vi "modeSuperposition_mk.vi"(0 "y_centre (in m; default 0)":dbl step=0.0001 format="%.5f", 1 "modes":T1(array[cluster])=[{"type"=enum."LG mode", "m or L"=-2, "n or p"=0, "weight"=0.7071, "phase"=0.0}, {"type"=enum."LG mode", "m or L"=2, "n or p"=0, "weight"=0.7071, "phase"=0.0}], 2 "beam waist w0 (in m; default 1E-4 = 0.1mm)":dbl=0.0005 format="%.2p", 3 "number of columns in amplitude matrix":i32, 4 "wavelength (in m)":dbl=7.1e-07 format="%#_6p", 5 "number of rows in amplitude matrix":i32, 6 "x_centre (in m; default 0)":dbl step=0.0001 format="%.5f", 8 "represented width & height (in m)":dbl=0.006 format="%#_6p") -> (7 "mode superposition":T2={"amplitude matrix"=array600x600[360000 elements], "number of columns in amplitude matrix"=600, "number of rows in amplitude matrix"=600, "represented width (in m)"=0.006, "represented height (in m)"=0.006, "wavelength (in m)"=7.1e-07})   [LabVIEW 2015]
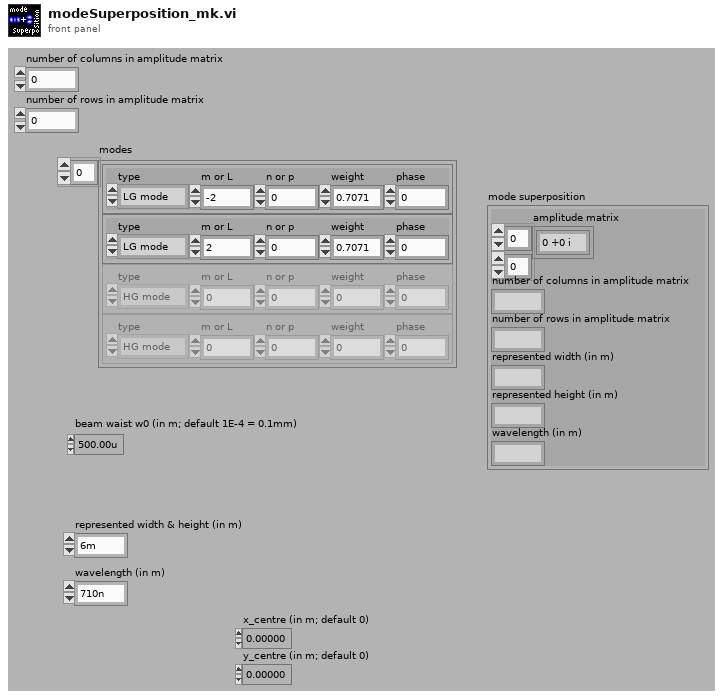
[diagram p1: front panel]
types:
  T1 = cluster{"type":enum16{"HG mode", "LG mode"}, "m or L":i32, "n or p":i32, "weight":dbl, "phase":dbl}[]
  T2 = cluster{"amplitude matrix":cdb[][], "number of columns in amplitude matrix":i32, "number of rows in amplitude matrix":i32, "represented width (in m)":dbl, "represented height (in m)":dbl, "wavelength (in m)":dbl}
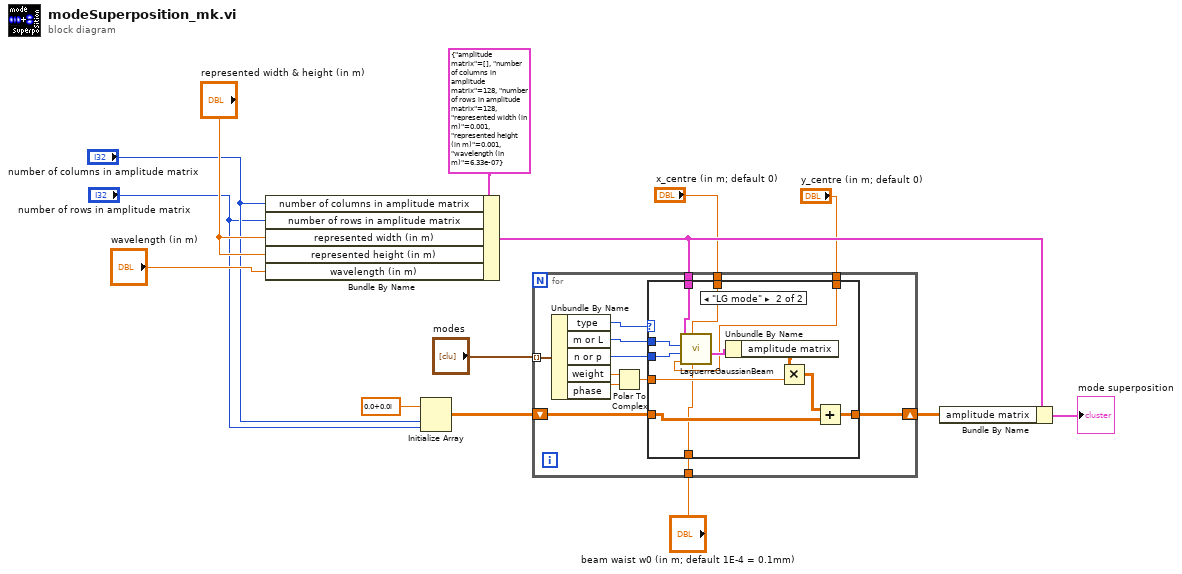
[diagram p0: block diagram]
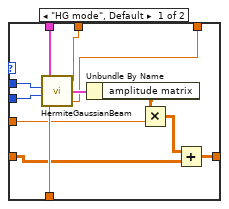
[diagram p2: hidden frame]
diagram:
  n1 = Bundle By Name(cluster=T2 {"amplitude matrix"=[], "number of columns in amplitude matrix"=128, "number of rows in amplitude matrix"=128, "represented width (in m)"=0.001, "represented height (in m)"=0.001, "wavelength (in m)"=6.33e-07} ("beam parameters"), "number of columns in amplitude matrix"="number of columns in amplitude matrix", "number of rows in amplitude matrix"="number of rows in amplitude matrix", "represented width (in m)"="represented width & height (in m)", "represented height (in m)"="represented width & height (in m)", "wavelength (in m)"="wavelength (in m)") -> (w7:T2)
  n2 = Initialize Array(cdb 0.0+0.0i ("element"), "number of columns in amplitude matrix", "number of rows in amplitude matrix") -> (w13:cdb[][])
  n3 = for {
    tunnel: "modes" -> [w27] mode=indexing
    shift-right: [w18] -> w8
    shift-left: w13 -> [w17]
    tunnel: w7 -> [w24]
    tunnel: "beam waist w0 (in m; default 1E-4 = 0.1mm)" -> [w25]
    tunnel: "x_centre (in m; default 0)" -> [w16]
    tunnel: "y_centre (in m; default 0)" -> [w15]
    n4 = Unbundle By Name(w27) -> ("type"=w26:enum16{"HG mode", "LG mode"}, "m or L"=w23:i32, "n or p"=w22:i32, "weight"=w21:dbl, "phase"=w20:dbl)
    n5 = Polar To Complex(1:w20, 2:w21) -> (0:w19:cdb)
    n6 = case shown="\"LG mode\"" w26 {
      tunnel: w25 -> [w39 w40]
      tunnel: w24 -> [w38 w51]
      tunnel: w23 -> [w37 w50]
      tunnel: w22 -> [w36 w49]
      tunnel: w19 -> [w33 w46]
      tunnel: [w32 w45] -> w18
      tunnel: w17 -> [w31 w44]
      tunnel: w16 -> [w29 w42]
      tunnel: w15 -> [w28 w41]
      frame "HG mode", Default {
        n7 = call <userlib>:"HermiteGaussianBeam.vi"("y_centre (in m; default 0)"=w28, "x_centre (in m; default 0)"=w29, "beam waist w0 (in m; default 1E-4 = 0.1mm)"=w39, "m"=w36, "n"=w37, "beam parameters"=w38) -> ("Hermite-Gaussian beam"=w35:T2)
        n8 = Unbundle By Name(w35) -> ("amplitude matrix"=w34:cdb[][])
        n9 = Multiply(x=w34, y=w33) -> (x*y=w30:cdb[][])
        n10 = Add(x=w30, y=w31) -> (x+y=w32:cdb[][])
      }
      frame "LG mode" {
        n11 = call <userlib>:"LaguerreGaussianBeam.vi"("beam waist w0 (in m; default 1E-4 = 0.1mm)"=w40, "x centre"=w42, "y centre"=w41, "p"=w49, "l"=w50, "beam parameters"=w51) -> ("Laguerre-Gaussian beam"=w48:T2)  [unwired: 5 in]
        n12 = Unbundle By Name(w48) -> ("amplitude matrix"=w47:cdb[][])
        n13 = Multiply(x=w47, y=w46) -> (x*y=w43:cdb[][])
        n14 = Add(x=w43, y=w44) -> (x+y=w45:cdb[][])
      }
    }
  }
  n15 = Bundle By Name(cluster=w7, "amplitude matrix"=w8) -> (→"mode superposition":T2)
